vi "testVi.vi"(1 "reference":refnum<vi>) -> (0 "Class Name 2":string)   [LabVIEW 2009]
panel:
  out "Value 2":variant
  out "Class Name":string
  out "Value":variant
  out "Unit Label.Text":string
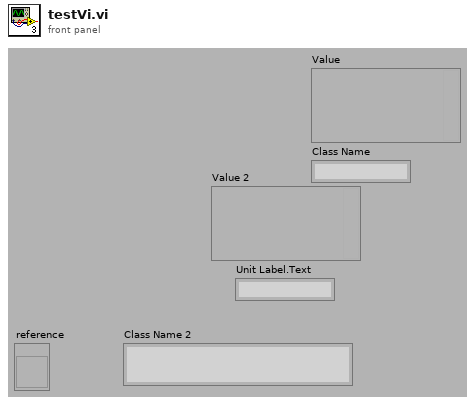
[diagram p1: front panel]
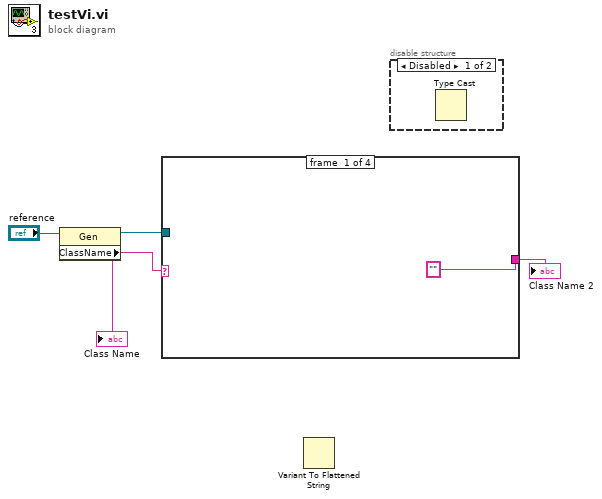
[diagram p0: block diagram]
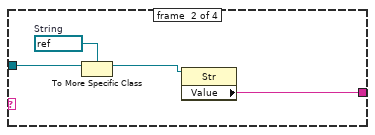
[diagram p3: hidden frame]
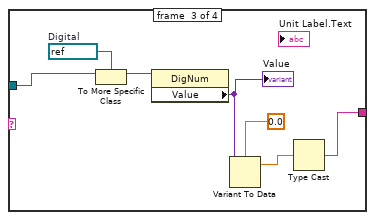
[diagram p4: hidden frame]
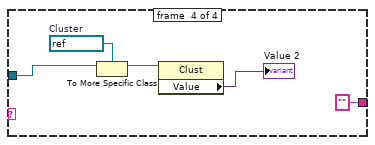
[diagram p5: hidden frame]
diagram:
  n1 = property class="Gen"(reference="reference") -> (reference out=w2:refnum<vi>, "ClassName"=w3:string)  [unwired: 1 in, 1 out]
  "Class Name" <- w3
  n2 = case shown="\"Cluster\"" w3 {
    tunnel: w2 -> [_ w7 w15 w18]
    tunnel: ["" ("Value") w9 w10 "" ("Value")] -> w1
    frame #0 {
    }
    frame #1 {
      w8 = refnum<vi> refnum  # String
      n3 = To More Specific Class(target class=w8, reference=w7) -> (specific class reference=w6:refnum<vi>)  [unwired: 1 in, 1 out]
      n4 = property class="Str"(reference=w6) -> ("Value"=w9:string)  [unwired: 1 in, 2 out]
    }
    frame #2 {
      w16 = refnum<vi> refnum  # Digital
      n5 = To More Specific Class(target class=w16, reference=w15) -> (specific class reference=w14:refnum<vi>)  [unwired: 1 in, 1 out]
      n6 = property class="DigNum"(reference=w14) -> ("Value"=w13:variant)  [unwired: 1 in, 2 out]
      "Value" <- w13
      n7 = Variant To Data(Variant=w13, type=0.0) -> (data=w11:dbl)  [unwired: 1 in, 1 out]
      n8 = Type Cast(x=w11) -> (*(type *) &x=w10:string)  [unwired: 1 in]
    }
    frame #3 {
      w21 = refnum<vi> refnum  # Cluster
      n9 = To More Specific Class(target class=w21, reference=w18) -> (specific class reference=w20:refnum<vi>)  [unwired: 1 in, 1 out]
      n10 = property class="Clust"(reference=w20) -> ("Value"=→"Value 2":variant)  [unwired: 1 in, 2 out]
    }
  }
  "Class Name 2" <- w1
  n11 = Variant To Flattened String() -> ()  [unwired: 1 in, 2 out]
  n12 = disable-structure shown="Disabled" {
    frame #0 {
      n13 = Type Cast() -> ()  [unwired: 2 in, 1 out]
    }
    frame #1 {
    }
  }
